vi "Build CSM to PPL.vi"(7 "Enable Conditional Building lvlibp?":bool=TRUE, 8 "error in":errorcluster) -> (0 "error out":errorcluster, 2 "Generated files":path[](array[path]))   [LabVIEW 2017]
uses:
  <vilib>/AppBuilder/AB_API_Simple/Build (path).vi
  <vilib>/AppBuilder/AB_API_Simple/NI_App_Builder_API.lvlib
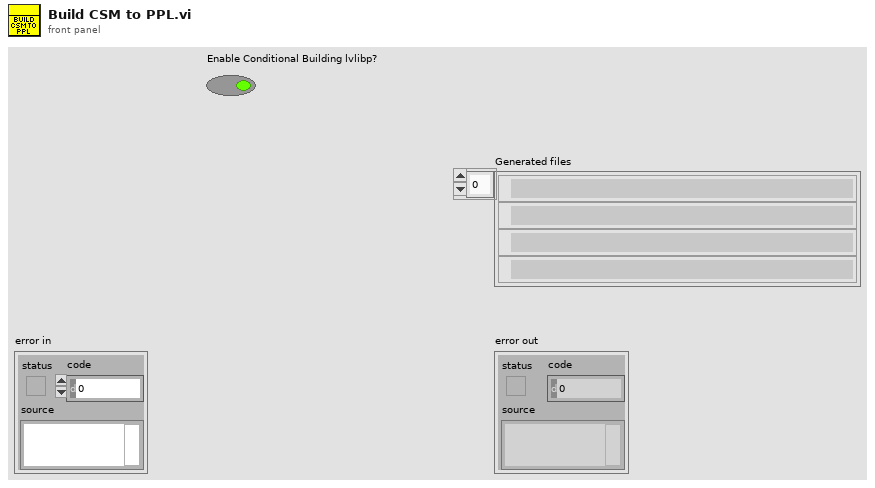
[diagram p1: front panel]
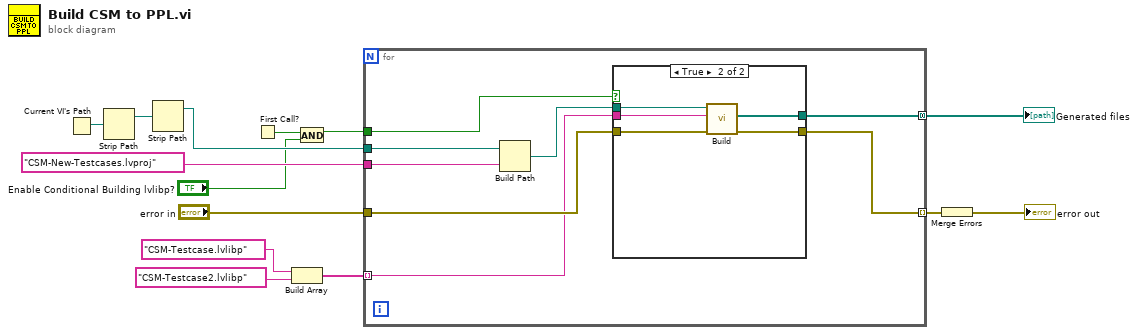
[diagram p0: block diagram]
diagram:
  n1 = Current VI's Path() -> (path=w11:path)
  n2 = Strip Path(path=w11) -> (stripped path=w12:path)  [unwired: 1 out]
  n3 = Strip Path(path=w12) -> (stripped path=w13:path)  [unwired: 1 out]
  n4 = First Call?() -> (First Call?: T/F=w4:bool)
  n5 = Build Array("CSM-Testcase.lvlibp" ("Name of build specification (if empty: build all)"), "CSM-Testcase2.lvlibp" ("Name of build specification (if empty: build all)")) -> (w7:string[])
  n6 = And(x=w4, y="Enable Conditional Building lvlibp?") -> (x .and. y?=w3:bool)
  n7 = for {
    tunnel: "CSM-New-Testcases.lvproj" ("name or relative path") -> [w21]
    tunnel: w13 -> [w20]
    tunnel: w7 -> [w19] mode=indexing
    tunnel: [w18] -> w6 mode=concatenating
    tunnel: w3 -> [w17]
    tunnel: "error in" -> [w22]
    tunnel: [w16] -> w10 mode=indexing
    n8 = Build Path(base path=w20, name or relative path=w21) -> (appended path=w15:path)
    n9 = case shown="True" w17 {
      tunnel: w22 -> [w23 w28]
      tunnel: [w23 w27] -> w16
      tunnel: w19 -> [_ w26]
      tunnel: [_ w25] -> w18
      tunnel: w15 -> [_ w24]
      frame False {
      }
      frame True {
        n10 = call-poly <vilib>:"Build.vi"("error in (no error)"=w28, "Name of build specification (if empty: build all)"=w26, "Path to project"=w24) -> ("error out"=w27:errorcluster, "Generated files"=w25:path[])  [unwired: 7 in]
      }
    }
  }
  "Generated files" <- w6
  n11 = Merge Errors(w10) -> (→"error out":errorcluster)
